vi "Read Target Data.vi"() -> (3 "Limilight Target Data":T1)   [LabVIEW 2019]
uses:
  <vilib>/Rock Robotics/Network Tables/NT Read Number.vi
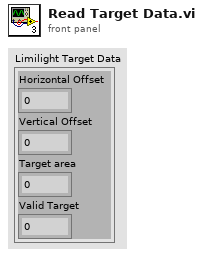
[diagram p1: front panel]
types:
  T1 = cluster{"Horizontal Offset":dbl, "Vertical Offset":dbl, "Target area":dbl, "Valid Target":dbl}
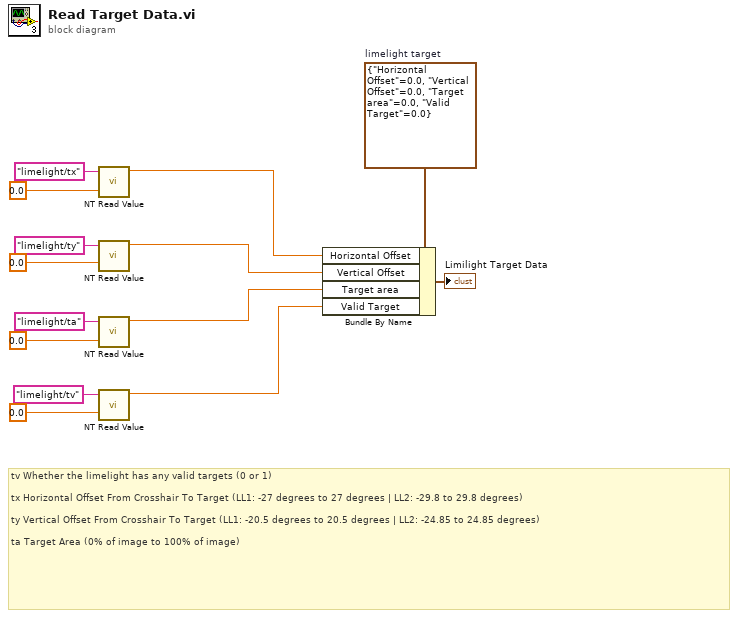
[diagram p0: block diagram]
diagram:
  w10 = T1 {"Horizontal Offset"=0.0, "Vertical Offset"=0.0, "Target area"=0.0, "Valid Target"=0.0}  # limelight target
  # "tv\tWhether the limelight has any valid targets (0 or 1)\n\ntx\tHorizontal Offset From Crosshair To Target (LL1: -27 degrees to 27 degrees | LL2: -29.8 to 29.8 degrees)\n\nty\tVertical Offset From Crosshair To Target (LL1: -20.5 degrees to 20.5 degrees | LL2: -24.85 to 24.85 degrees)\n\nta\tTarget Area (0% of image to 100% of image)"
  n1 = call-poly <vilib>:"NT Read Value.vi"("Default Value"=0.0, "Name"="limelight/tx") -> ("Numeric"=w9:dbl)  [unwired: 8 in, 1 out]
  n2 = call-poly <vilib>:"NT Read Value.vi"("Default Value"=0.0, "Name"="limelight/ty") -> ("Numeric"=w8:dbl)  [unwired: 8 in, 1 out]
  n3 = call-poly <vilib>:"NT Read Value.vi"("Default Value"=0.0, "Name"="limelight/ta") -> ("Numeric"=w7:dbl)  [unwired: 8 in, 1 out]
  n4 = call-poly <vilib>:"NT Read Value.vi"("Default Value"=0.0, "Name"="limelight/tv") -> ("Numeric"=w6:dbl)  [unwired: 8 in, 1 out]
  n5 = Bundle By Name(cluster=w10, "Horizontal Offset"=w9, "Vertical Offset"=w8, "Target area"=w7, "Valid Target"=w6) -> (→"Limilight Target Data":T1)
